vi "Assess Current Motor State.vi"(8 "error in (no error)":errorcluster, 11 "Elevator in":refnum<class "Elevator.lvclass">) -> (0 "error out":errorcluster, 3 "Elevator out":refnum<class "Elevator.lvclass">)   [LabVIEW 2014, in "Elevator.lvlib" / "Elevator.lvclass"]
uses:
  Elevator.lvclass
  Elevator State.ctl
  Elevator.lvclass/Elevator.ctl
  <vilib>/ActorFramework/Message Enqueuer/Message Enqueuer.lvclass/Message Enqueuer.ctl
  <vilib>/ActorFramework/Message Enqueuer/Enqueue.vi
  <vilib>/ActorFramework/Message Priority Queue/Priority Enqueue.vi
  Motor with Encoders/Motors with Encoders Messages/Zero Distance Msg/Zero Distance Msg.lvclass
panel:
  out "Elevator State":T1 {"Current Elevation" scale=0.0..100.0; "Current Travel Rate" scale=-1.0..1.0}
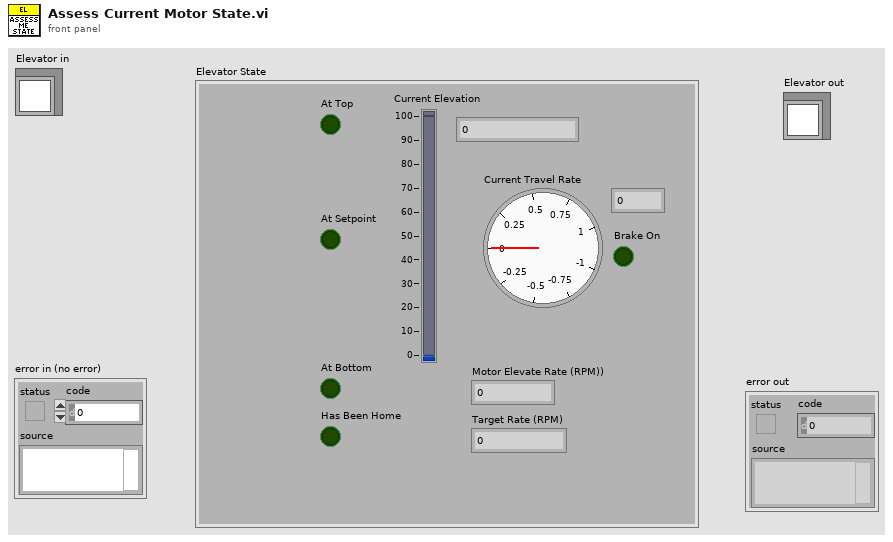
[diagram p1: front panel]
types:
  T1 = typedef "Elevator.lvlib/Elevator.lvclass/Elevator State.ctl" = cluster{"At Bottom":bool, "At Top":bool, "At Setpoint":bool, "Target Rate (RPM)":dbl, "Current Travel Rate":dbl, "Current Elevation":dbl, "Brake On":bool, "Motor Elevate Rate (RPM))":dbl, "Has Been Home":bool}
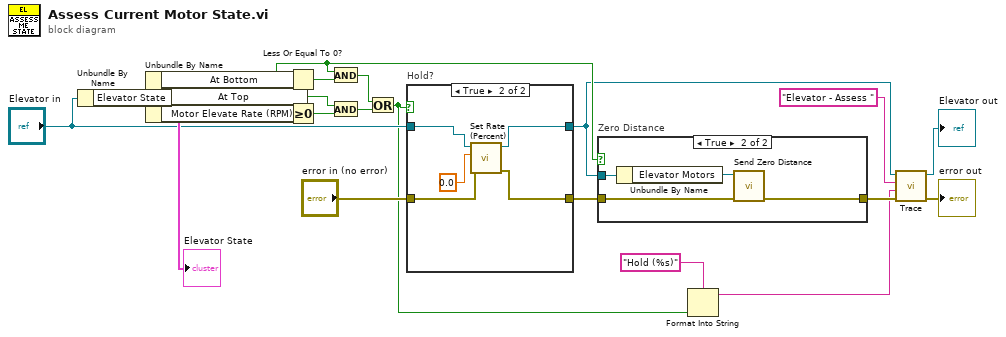
[diagram p0: block diagram]
diagram:
  n1 = Unbundle By Name("Elevator in") -> ("Elevator State"=w19:T1)
  "Elevator State" <- w19
  n2 = Unbundle By Name(w19) -> ("At Bottom"=w12:bool, "At Top"=w15:bool, "Motor Elevate Rate (RPM))"=w16:dbl)
  n3 = Less Or Equal To 0?(x=w16) -> (x <= 0?=w18:bool)
  n4 = Greater Or Equal To 0?(x=w16) -> (x >= 0?=w14:bool)
  n5 = And(x=w12, y=w18) -> (x .and. y?=w17:bool)
  n6 = And(x=w15, y=w14) -> (x .and. y?=w13:bool)
  n7 = Or(x=w17, y=w13) -> (x .or. y?=w1:bool)
  n8 = case "Hold?" shown="True" w1 {
    tunnel: "Elevator in" -> [w21 w26]
    tunnel: [w21 w25] -> w8
    tunnel: "error in (no error)" -> [w20 w23]
    tunnel: [w20 w22] -> w9
    frame False {
    }
    frame True {
      n9 = call-dynamic "Set Rate (Percent).vi"("error in (no error)"=w23, "Percent"=0.0 ("Rate"), "Elevator in"=w26) -> ("error out"=w22:errorcluster, "Elevator out"=w25:refnum<class "Elevator.lvclass">)  [unwired: 7 in]
    }
  }
  n10 = case "Zero Distance" shown="True" w12 {
    tunnel: w8 -> [_ w31]
    tunnel: w9 -> [w27 w29]
    tunnel: [w27 w28] -> w6
    frame False {
    }
    frame True {
      n11 = Unbundle By Name(w31) -> ("Elevator Motors"=w30:refnum<class "Message Enqueuer.lvclass">)
      n12 = call "Send Zero Distance.vi"("error in (no error)"=w29, "Message Enqueuer"=w30) -> ("error out"=w28:errorcluster)  [unwired: 8 in, 1 out]
    }
  }
  n13 = Format Into String(format string="Hold (%s)", w1) -> (resulting string=w2:string)  [unwired: 2 in, 1 out]
  n14 = call-dynamic "Trace.vi"("error in (no error)"=w6, "System Message"=w2, "System Action"="Elevator - Assess ", "System Actor in"=w8) -> ("error out"=→"error out":errorcluster, "System Actor out"=→"Elevator out":refnum<class "Elevator.lvclass">)  [unwired: 6 in]
